vi "Untitled 21 (SubVI).vi"(6 "gammag":dbl, 9 "Turbi. Eff.":dbl, 10 "T3t":dbl, 11 "Turbine prssure ratio":dbl) -> (3 "T4":dbl)   [LabVIEW 2019]
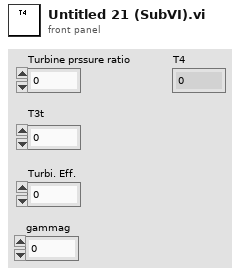
[diagram p1: front panel]
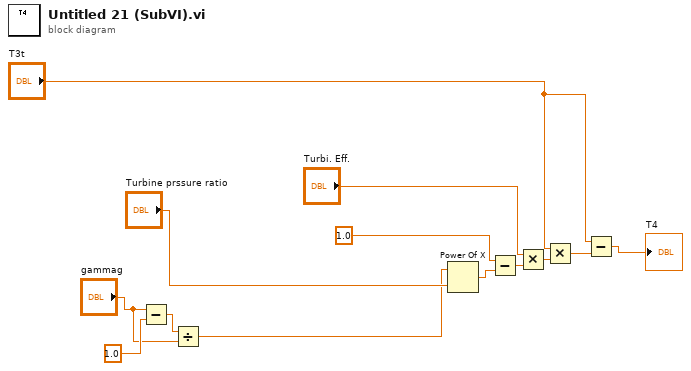
[diagram p0: block diagram]
diagram:
  n1 = Subtract(x="gammag", y=1.0) -> (x-y=w12:dbl)
  n2 = Divide(x=w12, y="gammag") -> (x/y=w9:dbl)
  n3 = Power Of X(1:"Turbine prssure ratio", 2:w9) -> (0:w8:dbl)
  n4 = Subtract(x=1.0, y=w8) -> (x-y=w6:dbl)
  n5 = Multiply(x="Turbi. Eff.", y=w6) -> (x*y=w4:dbl)
  n6 = Multiply(x="T3t", y=w4) -> (x*y=w3:dbl)
  n7 = Subtract(x="T3t", y=w3) -> (x-y=→"T4":dbl)
